vi "Acquire Single Image (Snap).vi"() -> ()   [LabVIEW 2023]
doc: "The Acquire Single Image (Snap) example acquires an image and displays the image in an image control. A snap is appropriate for low-speed or single-capture applications in which ease of programming is essential."
uses:
  <vilib>/vision/driver/NI_Vision_Acquisition_Software.lvlib
panel:
  in  "Camera Name":refnum<k21> caption="IMAQdx Session"
  out "Image":T1(plugin-control)
  # "Overview: Demonstrates how to acquire a single image.\nRequirements: Vision Acquisition Software\nInstructions: \n1. Select the Camera Name.\n2. Run the VI"
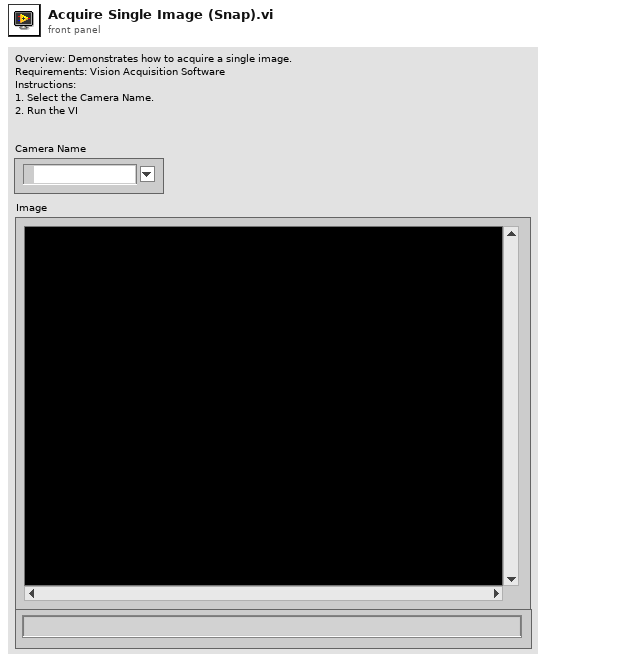
[diagram p1: front panel]
types:
  T1 = typedef "IMAQ Image.ctl" = refnum<image>
  T2 = typedef "IMAQdx.ctl" = refnum<k21>
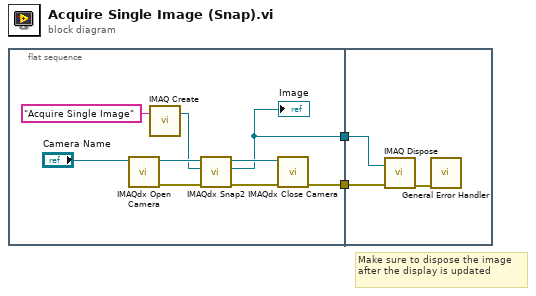
[diagram p0: block diagram]
diagram:
  # "Make sure to dispose the image after the display is updated"
  n1 = flat-sequence {
    tunnel: [w10] -> w2
    tunnel: [w3] -> w1
    tunnel: w2 -> [w14]
    tunnel: w1 -> [w13]
    frame #0 {
      n2 = call <vilib>:"IMAQdx Open Camera.vi"("Session In"="Camera Name") -> ("error out"=w6:errorcluster, "Session Out"=w9:T2)  [unwired: 2 in, 7 out]
      n3 = call "IMAQ Create"("Image Name"="Acquire Single Image") -> ("New Image"=w5:T1)  [unwired: 3 in, 2 out]
      n4 = call <vilib>:"IMAQdx Snap2.vi"("error in"=w6, "Image In"=w5, "Session In"=w9) -> ("error out"=w8:errorcluster, "Image Out"=w3:T1, "Session Out"=w11:T2)  [unwired: 6 in]
      "Image" <- w3
      n5 = call <vilib>:"IMAQdx Close Camera.vi"("error in"=w8, "Session In"=w11) -> ("error out"=w10:errorcluster)  [unwired: 9 out]
    }
    frame #1 {
      n6 = call "IMAQ Dispose"("Image"=w13, "error in (no error)"=w14) -> ("error out"=w12:errorcluster)  [unwired: 4 in]
      n7 = call <vilib>:"General Error Handler.vi"("error in (no error)"=w12) -> ()  [unwired: 2 in, 13 out]
    }
  }
